vi "TestEnsureIgorStringFormat.vi"(8 "error in (no error)":errorcluster) -> (0 "error out":errorcluster)   [LabVIEW 2019]
uses:
  <vilib>/addons/_JKI Toolkits/Caraya/classes/Test/Test.lvclass
  <vilib>/addons/_JKI Toolkits/Caraya/classes/Assert/Assert.lvclass
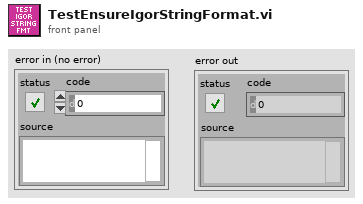
[diagram p1: front panel]
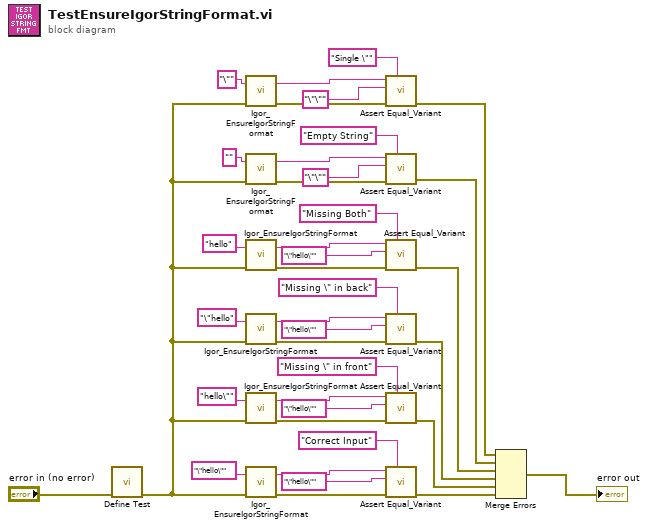
[diagram p0: block diagram]
diagram:
  n1 = call <vilib>:"Define Test.vi"("error in (no error)"="error in (no error)") -> ("error out"=w1:errorcluster)  [unwired: 10 in]
  n2 = call "Igor_EnsureIgorStringFormat.vi"("Value"="\"") -> ("Value"=w3:string)  [unwired: 2 in]
  n3 = call "Igor_EnsureIgorStringFormat.vi"("Value"="") -> ("Value"=w10:string)  [unwired: 2 in]
  n4 = call "Igor_EnsureIgorStringFormat.vi"("Value"="hello") -> ("Value"=w21:string)  [unwired: 2 in]
  n5 = call "Igor_EnsureIgorStringFormat.vi"("Value"="\"hello") -> ("Value"=w14:string)  [unwired: 2 in]
  n6 = call "Igor_EnsureIgorStringFormat.vi"("Value"="hello\"") -> ("Value"=w23:string)  [unwired: 2 in]
  n7 = call "Igor_EnsureIgorStringFormat.vi"("Value"="\"hello\"") -> ("Value"=w30:string)  [unwired: 2 in]
  n8 = call <vilib>:"Assert Equal_Variant.vi"("Label"="Single \"", "error in (no error)"=w1, "Y"="\"\"" ("Label"), "X"=w3) -> ("error out"=w2:errorcluster)  [unwired: 7 in]
  n9 = call <vilib>:"Assert Equal_Variant.vi"("Label"="Empty String", "error in (no error)"=w1, "Y"="\"\"" ("Label"), "X"=w10) -> ("error out"=w11:errorcluster)  [unwired: 7 in]
  n10 = call <vilib>:"Assert Equal_Variant.vi"("Label"="Missing Both", "error in (no error)"=w1, "Y"="\"hello\"" ("Value"), "X"=w21) -> ("error out"=w12:errorcluster)  [unwired: 7 in]
  n11 = call <vilib>:"Assert Equal_Variant.vi"("Label"="Missing \" in back", "error in (no error)"=w1, "Y"="\"hello\"" ("Value"), "X"=w14) -> ("error out"=w13:errorcluster)  [unwired: 7 in]
  n12 = call <vilib>:"Assert Equal_Variant.vi"("Label"="Missing \" in front", "error in (no error)"=w1, "Y"="\"hello\"" ("Value"), "X"=w23) -> ("error out"=w22:errorcluster)  [unwired: 7 in]
  n13 = call <vilib>:"Assert Equal_Variant.vi"("Label"="Correct Input", "error in (no error)"=w1, "Y"="\"hello\"" ("Value"), "X"=w30) -> ("error out"=w31:errorcluster)  [unwired: 7 in]
  n14 = Merge Errors(w2, w11, w12, w13, w22, w31) -> (→"error out":errorcluster)
